vi "Inst.Attocube-3DR.GetAllData.vi"(8 "error in (no error)":errorcluster, 11 "Inst.Attocube-3DR in":refnum<class "Inst.Attocube-3DR.lvclass">) -> (0 "error out":errorcluster, 2 "Data out":variant, 3 "Inst.Attocube-3DR out":refnum<class "Inst.Attocube-3DR.lvclass">)   [LabVIEW 2019, in "Inst.Attocube-3DR.lvclass"]
uses:
  Inst.Attocube-3DR.lvclass
  Typedefs/Inst.Attocube-3DR.getAll--Cluster.ctl
  Inst.Attocube-3DR.lvclass/Inst.Attocube-3DR.ctl
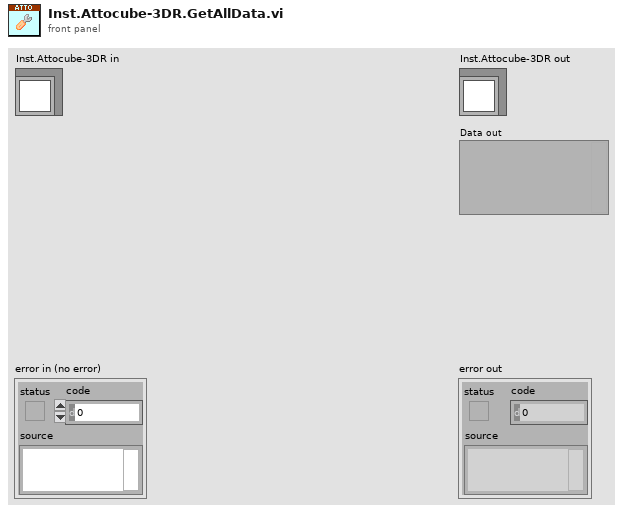
[diagram p1: front panel]
types:
  T1 = typedef "Inst.Attocube-3DR.lvclass/Inst.Attocube-3DR.getAll--Cluster.ctl" = cluster{"Axis 1: Amplitude":i32, "Axis 1: Capacitance":i32, "Axis 1: Current Position":i32, "Axis 1: DCLevel":i32, "Axis 1: Frequency":i32, "Axis 1: StepWidth":i32, "Axis 1: control mode":i32, "Axis 1: rot. count":i32, "Axis 1: sp position":i32, "Axis 1: sp rot. count":i32, "Axis 1: speed":i32, "Axis 1: Target GND":bool, "Axis 1: Output":bool, "Axis 1: Single Circle Mode":bool, "Axis 1: moving":bool, "Axis 1: stop detected":bool, "Axis 1:  sensor error":bool, "Axis 1: sensor diconnected":bool, "Axis 1: stop enable":bool, "Axis 2: Current Position":i32, "Axis 2: DCLevel":i32, "Axis 2: Frequency":i32, "Axis 2: StepWidth":i32, "Axis 2: control mode":i32, "Axis 2: rot. count":i32, "Axis 2: sp position":i32, "Axis 2: sp rot. count":i32, "Axis 2: speed":i32, "Axis 2: Capacitance":i32, "Axis 2: Amplitude":i32, "Axis 2: Target GND":bool, "Axis 2: Output":bool, "Axis 2: Single Circle Mode":bool, "Axis 2: moving":bool, "Axis 2: stop detected":bool, "Axis 2:  sensor error":bool, "Axis 2: sensor diconnected":bool, "Axis 2: stop enable":bool}
  T2 = cluster{"error ":bool, "error number":i32, "error code":string}
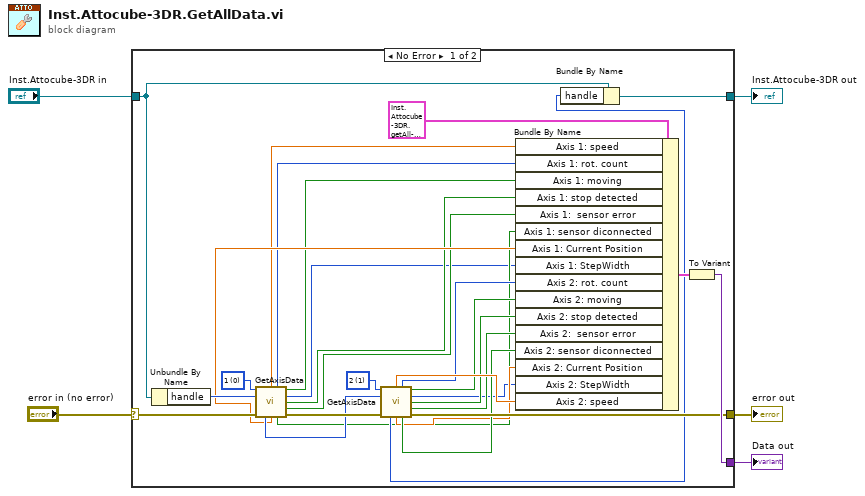
[diagram p0: block diagram]
diagram:
  n1 = case shown="No Error" "error in (no error)" {
    selector: "error in (no error)" -> [w26 w36]
    tunnel: [w25 w36] -> w5
    tunnel: [w34 w35] -> w3
    tunnel: "Inst.Attocube-3DR in" -> [w33 w35]
    tunnel: [w32 _] -> w2
    frame No Error {
      w28 = u8 1 items=["1", "2", "3", "4", "5", "6", "7", "8", "9"] ("axis no")
      w29 = u8 0 items=["1", "2", "3", "4", "5", "6", "7", "8", "9"] ("axis no")
      n2 = Unbundle By Name(w33) -> ("handle"=w24:i32)
      n3 = call "GetAxisData.vi"("axis no"=w29, "device handle"=w24, "error in (no error)"=w26) -> ("speed (°/s)"=w6:dbl, "count"=w7:i32, "moving"=w8:bool, "StepWidth"=w9:i32, "stop detected"=w10:bool, "sensor error"=w11:bool, "device handle 2"=w14:i32, "position [µm/°/m°]"=w13:dbl, "sensor disconnected"=w12:bool, "error out"=w27:T2)  [unwired: 3 in]
      n4 = call "GetAxisData.vi"("axis no"=w28, "device handle"=w14, "error in (no error)"=w27) -> ("speed (°/s)"=w22:dbl, "count"=w16:i32, "moving"=w21:bool, "StepWidth"=w15:i32, "stop detected"=w20:bool, "sensor error"=w19:bool, "device handle 2"=w23:i32, "position [µm/°/m°]"=w17:dbl, "sensor disconnected"=w18:bool, "error out"=w25:T2)  [unwired: 3 in]
      n5 = Bundle By Name(cluster=T1 {"Axis 1: Amplitude"=0, "Axis 1: Capacitance"=0, "Axis 1: Current Position"=0, "Axis 1: DCLevel"=0, "Axis 1: Frequency"=0, "Axis 1: StepWidth"=0, "Axis 1: control mode"=0, "Axis 1: rot. count"=0, "Axis 1: sp position"=0, "Axis 1: sp rot. count"=0, "Axis 1: speed"=0, "Axis 1: Target GND"=FALSE, "Axis 1: Output"=FALSE, "Axis 1: Single Circle Mode"=FALSE, "Axis 1: moving"=FALSE, "Axis 1: stop detected"=FALSE, "Axis 1:  sensor error"=FALSE, "Axis 1: sensor diconnected"=FALSE, "Axis 1: stop enable"=FALSE, "Axis 2: Current Position"=0, "Axis 2: DCLevel"=0, "Axis 2: Frequency"=0, "Axis 2: StepWidth"=0, "Axis 2: control mode"=0, "Axis 2: rot. count"=0, "Axis 2: sp position"=0, "Axis 2: sp rot. count"=0, "Axis 2: speed"=0, "Axis 2: Capacitance"=0, "Axis 2: Amplitude"=0, "Axis 2: Target GND"=FALSE, "Axis 2: Output"=FALSE, "Axis 2: Single Circle Mode"=FALSE, "Axis 2: moving"=FALSE, "Axis 2: stop detected"=FALSE, "Axis 2:  sensor error"=FALSE, "Axis 2: sensor diconnected"=FALSE, "Axis 2: stop enable"=FALSE} ("getAll"), "Axis 1: speed"=w6, "Axis 1: rot. count"=w7, "Axis 1: moving"=w8, "Axis 1: stop detected"=w10, "Axis 1:  sensor error"=w11, "Axis 1: sensor diconnected"=w12, "Axis 1: Current Position"=w13, "Axis 1: StepWidth"=w9, "Axis 2: rot. count"=w16, "Axis 2: moving"=w21, "Axis 2: stop detected"=w20, "Axis 2:  sensor error"=w19, "Axis 2: sensor diconnected"=w18, "Axis 2: Current Position"=w17, "Axis 2: StepWidth"=w15, "Axis 2: speed"=w22) -> (w31:T1)
      n6 = Bundle By Name(cluster=w33, "handle"=w23) -> (w34:refnum<class "Inst.Attocube-3DR.lvclass">)
      n7 = To Variant(anything=w31) -> (Variant=w32:variant)
    }
    frame Error {
    }
  }
  "error out" <- w5
  "Inst.Attocube-3DR out" <- w3
  "Data out" <- w2
